vi "calibratePlatformsAppended.vi"() -> ()   [LabVIEW 2017]
doc: "The load cells output a voltage even when no weight is present on the platform. This needs to be measured so that it can be subtracted from subsequent measurements of platform load. The VI will output a spreadsheet saved in the current folder."
uses:
  <vilib>/Utility/file.llb/Write Delimited Spreadsheet (DBL).vi
  <vilib>/Utility/file.llb/Write Delimited Spreadsheet (string).vi
panel:
  in  "mazeDirection":string(combo)="clockwise"
  out "Separated inputs\nas strings":string[](array[string])
  in  "platforms":i32[](array[numeric])
  out "x/y":dbl[](array[numeric])
  in  "stop 2":bool
  in  "50 g":bool
  in  "Zero":bool
  # "1. First zero the platforms\n2. Place 50 g weights on platforms\n3. Run 50 g calibration"
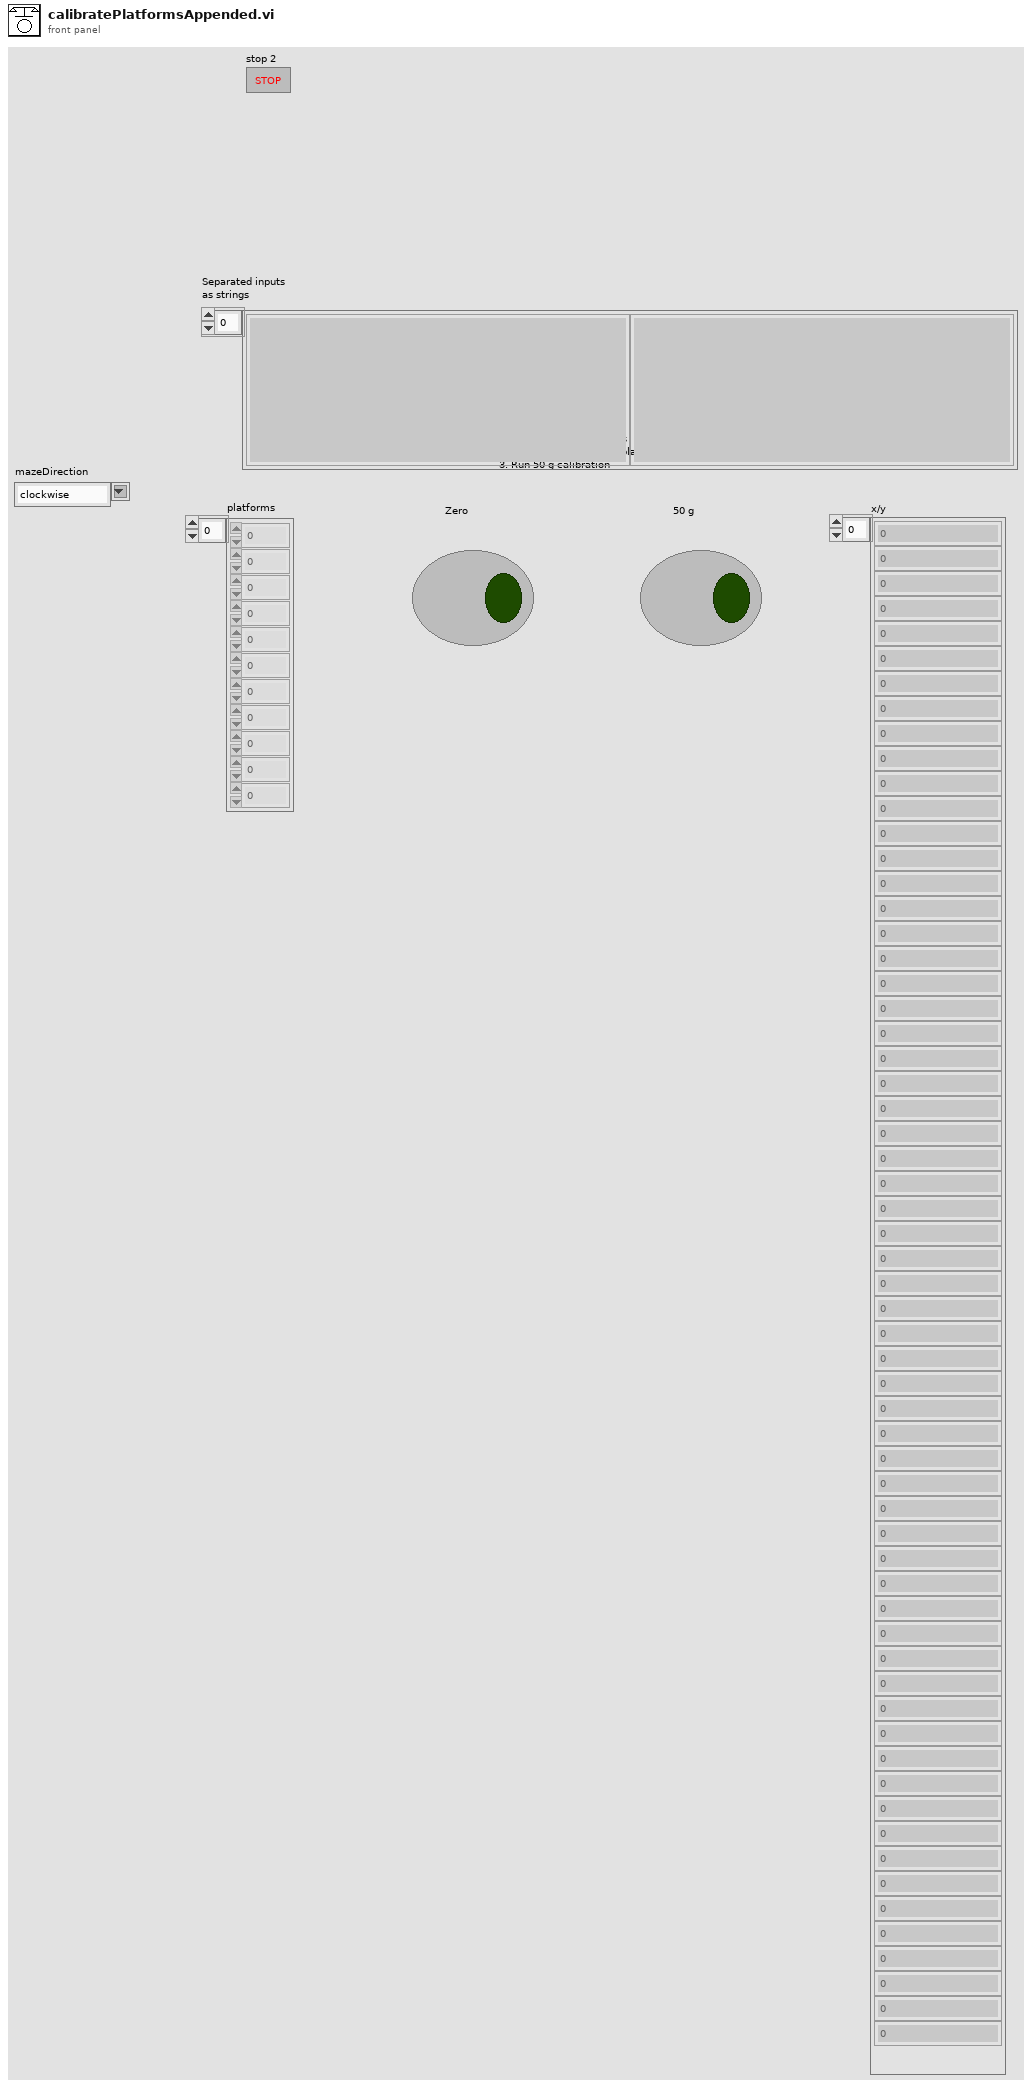
[diagram p1: front panel]
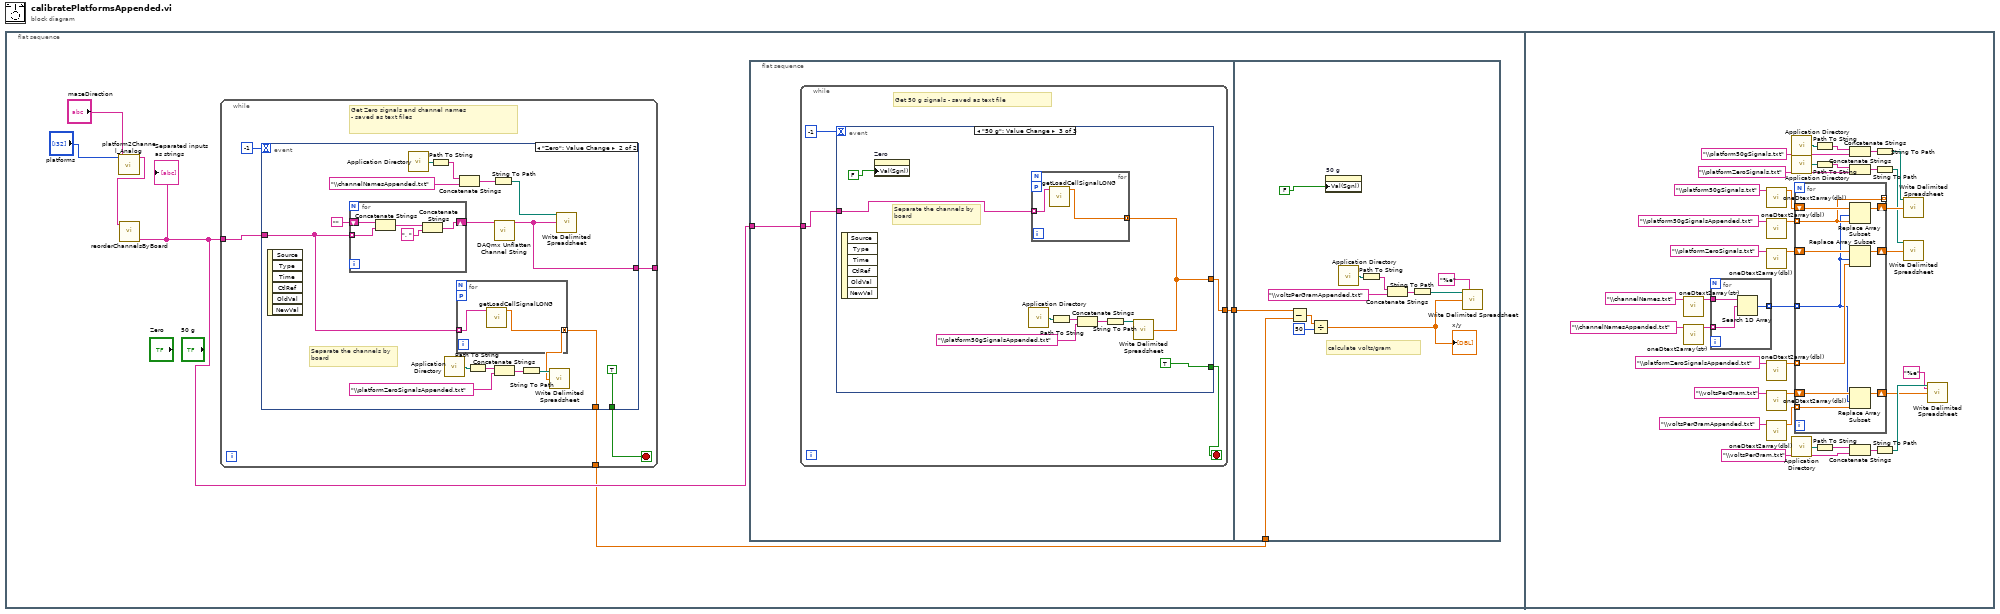
[diagram p0: block diagram]
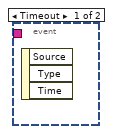
[diagram p2: hidden frame]
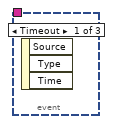
[diagram p3: hidden frame]
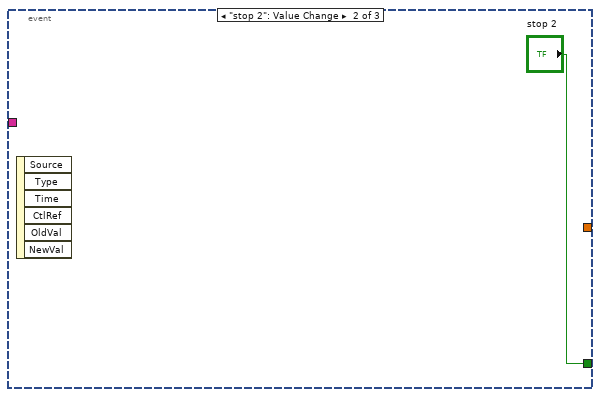
[diagram p4: hidden frame]
diagram:
  n1 = flat-sequence {
    frame #0 {
      n2 = call "platform2Channel_Analog.vi"("mazeDirection"="mazeDirection", "platforms"="platforms") -> ("DAQmx Channel"=w2:string)  [unwired: 9 in]
      n3 = call "reorderChannelsByBoard.vi"("DAQmx \nPhysical Channel"=w2) -> ("Separated inputs\nas strings"=w5:string[])  [unwired: 8 in, 2 out]
      "Separated inputs\nas strings" <- w5
      n4 = while {
        tunnel: w5 -> [w10]
        tunnel: [w8] -> w4
        tunnel: [w7] -> _
        stop <- w9 stop-if-true
        # "Get Zero signals and channel names \n- saved as text files"
        n5 = event shown="[1] \"Zero\": Value Change" {
          selector: _ -> [_ _]
          dyn-events: _ -> [_ _]
          timeout: -1 -> [_ _]
          tunnel: w10 -> [_ w15]
          tunnel: [_ w14] -> w8
          tunnel: [_ TRUE] -> w9
          tunnel: [_ w12] -> w7
          event Timeout {
            n6 = event-data() -> ()  [unwired: 1 in, 3 out]
          }
          event "Zero": Value Change {
            # "Separate the channels by\nboard"
            n7 = event-data() -> ()  [unwired: 1 in, 6 out]
            n8 = for {
              shift-right: [w31] -> w26
              shift-left: "" -> [w32]
              tunnel: w15 -> [w28] mode=indexing
              n9 = Concatenate Strings(w32, w28) -> (w30:string)
              n10 = Concatenate Strings(w30, ", ") -> (w31:string)
            }
            n11 = call <vilib>:"Application Directory.vi"() -> ("Application Directory"=w24:path)
            n12 = Path To String(path=w24) -> (string=w23:string)
            n13 = call <vilib>:"Application Directory.vi"() -> ("Application Directory"=w19:path)
            n14 = for {
              workers-P: _ -> [_]
              tunnel: [w33] -> w14 mode=concatenating
              tunnel: w15 -> [w34] mode=indexing
              n15 = call "getLoadCellSignalLONG.vi"("DAQmx Physical Channel"=w34) -> ("load cell\nsignal"=w33:dbl[])  [unwired: 10 in]
            }
            n16 = Concatenate Strings(w23, "\\channelNamesAppended.txt") -> (w22:string)
            n17 = Path To String(path=w19) -> (string=w18:string)
            n18 = String To Path(string=w22) -> (path=w21:path)
            n19 = call <vilib>:"DAQmx Unflatten Channel String.vi"("names in"=w26) -> ("names out"=w12:string[])  [unwired: 13 in, 1 out]
            n20 = Concatenate Strings(w18, "\\platformZeroSignalsAppended.txt") -> (w17:string)
            n21 = String To Path(string=w17) -> (path=w16:path)
            n22 = call-poly <vilib>:"Write Delimited Spreadsheet.vi"("file path (dialog if empty)"=w16, "1D data"=w14) -> ()  [unwired: 12 in, 2 out]
            n23 = call-poly <vilib>:"Write Delimited Spreadsheet.vi"("file path (dialog if empty)"=w21, "1D data"=w12) -> ()  [unwired: 12 in, 2 out]
          }
        }
      }
      n24 = flat-sequence {
        tunnel: w5 -> [w35]
        tunnel: [w36] -> w6
        tunnel: w6 -> [w54]
        tunnel: w4 -> [w55]
        frame #0 {
          n25 = while {
            tunnel: [w39] -> w36
            tunnel: w35 -> [w37]
            stop <- w38 stop-if-true
            # "Get 50 g signals - saved as text file"
            n26 = event shown="[2] \"50 g\": Value Change" {
              selector: _ -> [_ _ _]
              dyn-events: _ -> [_ _ _]
              timeout: -1 -> [_ _ _]
              tunnel: [_ "stop 2" TRUE] -> w38
              tunnel: [_ _ w44] -> w39
              tunnel: w37 -> [_ _ w42]
              event Timeout {
                n27 = event-data() -> ()  [unwired: 1 in, 3 out]
              }
              event "stop 2": Value Change {
                n28 = event-data() -> ()  [unwired: 1 in, 6 out]
              }
              event "50 g": Value Change {
                # "Separate the channels by\nboard"
                n29 = event-data() -> ()  [unwired: 1 in, 6 out]
                n30 = property on="Zero" class="Bool (strict)"("Val(Sgnl)"=FALSE) -> ()  [unwired: 2 in, 2 out]
                n31 = call <vilib>:"Application Directory.vi"() -> ("Application Directory"=w49:path)
                n32 = for {
                  workers-P: _ -> [_]
                  tunnel: [w51] -> w44 mode=concatenating
                  tunnel: w42 -> [w52] mode=indexing
                  n33 = call "getLoadCellSignalLONG.vi"("DAQmx Physical Channel"=w52) -> ("load cell\nsignal"=w51:dbl[])  [unwired: 10 in]
                }
                n34 = Path To String(path=w49) -> (string=w48:string)
                n35 = Concatenate Strings(w48, "\\platform50gSignalsAppended.txt") -> (w47:string)
                n36 = String To Path(string=w47) -> (path=w46:path)
                n37 = call-poly <vilib>:"Write Delimited Spreadsheet.vi"("file path (dialog if empty)"=w46, "1D data"=w44) -> ()  [unwired: 12 in, 2 out]
              }
            }
          }
        }
        frame #1 {
          # "calculate volts/gram"
          n38 = Subtract(x=w54, y=w55) -> (x-y=w59:dbl[])
          n39 = Divide(x=w59, y=50) -> (x/y=w64:dbl[])
          "x/y" <- w64
          n40 = property on="50 g" class="Bool (strict)"("Val(Sgnl)"=FALSE) -> ()  [unwired: 2 in, 2 out]
          n41 = call <vilib>:"Application Directory.vi"() -> ("Application Directory"=w60:path)
          n42 = Path To String(path=w60) -> (string=w61:string)
          n43 = Concatenate Strings(w61, "\\voltsPerGramAppended.txt") -> (w62:string)
          n44 = String To Path(string=w62) -> (path=w63:path)
          n45 = call-poly <vilib>:"Write Delimited Spreadsheet.vi"("file path (dialog if empty)"=w63, "format (%.3f)"="%e", "1D data"=w64) -> ()  [unwired: 11 in, 2 out]
        }
      }
    }
    frame #1 {
      n46 = call "oneDtext2array(str).vi"("String"="\\channelNames.txt") -> ("text"=w97:string[])  [unwired: 10 in]
      n47 = call "oneDtext2array(str).vi"("String"="\\channelNamesAppended.txt") -> ("text"=w98:string[])  [unwired: 10 in]
      n48 = for {
        tunnel: w98 -> [w112] mode=indexing
        tunnel: w97 -> [w113]
        tunnel: [w111] -> w92 mode=indexing
        n49 = Search 1D Array(1D array=w113, element=w112) -> (index of element=w111:i32)  [unwired: 1 in]
      }
      n50 = call "oneDtext2array(dbl).vi"("String"="\\platform50gSignals.txt") -> ("array"=w79:dbl[])  [unwired: 10 in]
      n51 = call "oneDtext2array(dbl).vi"("String"="\\platform50gSignalsAppended.txt") -> ("array"=w78:dbl[])  [unwired: 10 in]
      n52 = call "oneDtext2array(dbl).vi"("String"="\\platformZeroSignals.txt") -> ("array"=w89:dbl[])  [unwired: 10 in]
      n53 = call "oneDtext2array(dbl).vi"("String"="\\platformZeroSignalsAppended.txt") -> ("array"=w91:dbl[])  [unwired: 10 in]
      n54 = call "oneDtext2array(dbl).vi"("String"="\\voltsPerGram.txt") -> ("array"=w88:dbl[])  [unwired: 10 in]
      n55 = call "oneDtext2array(dbl).vi"("String"="\\voltsPerGramAppended.txt") -> ("array"=w90:dbl[])  [unwired: 10 in]
      n56 = call <vilib>:"Application Directory.vi"() -> ("Application Directory"=w76:path)
      n57 = call <vilib>:"Application Directory.vi"() -> ("Application Directory"=w70:path)
      n58 = call <vilib>:"Application Directory.vi"() -> ("Application Directory"=w86:path)
      n59 = for {
        tunnel: w92 -> [w102] mode=indexing
        tunnel: w91 -> [w105] mode=indexing
        tunnel: w90 -> [w110] mode=indexing
        shift-right: [w109] -> w82
        shift-left: w88 -> [w108]
        shift-right: [w106] -> w66
        shift-left: w89 -> [w107]
        shift-right: [w101] -> w72
        shift-left: w79 -> [w104]
        tunnel: [w103] -> _ mode=indexing
        tunnel: w78 -> [w103] mode=indexing
        n60 = Replace Array Subset(array=w104, new element=w103, index=w102) -> (w101:dbl[])
        n61 = Replace Array Subset(array=w107, new element=w105, index=w102) -> (w106:dbl[])
        n62 = Replace Array Subset(array=w108, new element=w110, index=w102) -> (w109:dbl[])
      }
      n63 = Path To String(path=w76) -> (string=w75:string)
      n64 = Path To String(path=w70) -> (string=w69:string)
      n65 = Path To String(path=w86) -> (string=w85:string)
      n66 = Concatenate Strings(w75, "\\platform50gSignals.txt") -> (w74:string)
      n67 = Concatenate Strings(w69, "\\platformZeroSignals.txt") -> (w68:string)
      n68 = Concatenate Strings(w85, "\\voltsPerGram.txt") -> (w84:string)
      n69 = String To Path(string=w74) -> (path=w73:path)
      n70 = String To Path(string=w68) -> (path=w67:path)
      n71 = String To Path(string=w84) -> (path=w83:path)
      n72 = call-poly <vilib>:"Write Delimited Spreadsheet.vi"("file path (dialog if empty)"=w73, "1D data"=w72) -> ()  [unwired: 12 in, 2 out]
      n73 = call-poly <vilib>:"Write Delimited Spreadsheet.vi"("file path (dialog if empty)"=w67, "1D data"=w66) -> ()  [unwired: 12 in, 2 out]
      n74 = call-poly <vilib>:"Write Delimited Spreadsheet.vi"("file path (dialog if empty)"=w83, "format (%.3f)"="%e", "1D data"=w82) -> ()  [unwired: 11 in, 2 out]
    }
  }
